vi "ExampleQueueSize.vi"() -> ()   [LabVIEW 2016]
uses:
  AdvancedDataStructures/ClassBased/Applications/PriorityQueue/PriorityQueue/PriorityQueue.lvclass
  AdvancedDataStructures/ClassBased/LinkedList/LinkedList.lvclass
panel:
  out "size":i32
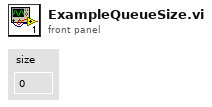
[diagram p1: front panel]
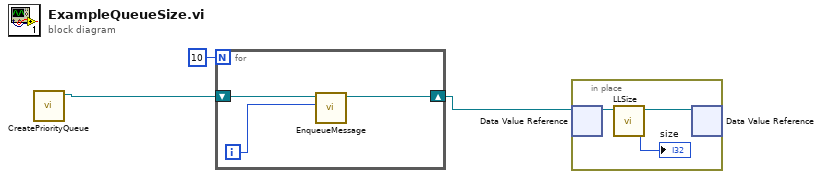
[diagram p0: block diagram]
diagram:
  n1 = call "CreatePriorityQueue.vi"() -> ("PriorityQueue"=w3:refnum<data-value>)  [unwired: 10 in, 1 out]
  n2 = for {
    N: 10 -> [_]
    shift-right: [w4] -> w2
    shift-left: w3 -> [w5]
    i -> [w6]
    n3 = call "EnqueueMessage.vi"("message"=w6, "queue in"=w5) -> ("queue out"=w4:refnum<data-value>)  [unwired: 8 in, 1 out]
  }
  n4 = in-place {
    n5 = in-place-dvr #1(w2) -> (w9:refnum<class "PriorityQueue.lvclass">)  [unwired: 1 out]
    n6 = call "LLSize.vi"("LinkedList in"=w9) -> ("size"=→"size":i32, "LinkedList out"=w8:refnum<class "PriorityQueue.lvclass">)  [unwired: 8 in, 1 out]
    n7 = in-place-dvr #1(w8) -> ()  [unwired: 2 out]
  }
